vi "Lab Panel V4.89.vi"() -> ()   [LabVIEW 2013] (continued)
                            n1479 = local write "RESULT LAB05-2"(TRUE) -> ()
                            n1480 = local write "DISP LAB05-2"(w2793) -> ()
                          }
                        }
                      }
                      frame False {
                      }
                    }
                  }
                }
              }
            }
          }
          frame #6 {
            # "end test & close test files"
            n1481 = local read "MAIL SETTINGS"() -> (w2799:T7)
            n1482 = Unbundle(w2799) -> ("OUT SERVER ADDRESS"=w2798:string, "FROM ACCOUNT"=w2797:string)  [unwired: 5 out]
            n1483 = stacked-sequence {
              tunnel: w2809 -> [_ _ _ _ _ _ _ _ _ _]
              tunnel: w2810 -> [_ _ _ _ _ _ _ _ _ _]
              tunnel: w2808 -> [_ _ _ _ _ _ _ _ _ _]
              tunnel: w2807 -> [_ _ _ _ _ _ _ _ _ _]
              tunnel: w2806 -> [_ _ _ _ _ _ _ _ _ _]
              tunnel: w2805 -> [_ _ _ _ _ _ _ _ _ _]
              tunnel: w2804 -> [_ _ _ _ _ _ _ _ _ _]
              tunnel: w2803 -> [_ _ _ _ _ _ _ _ _ _]
              tunnel: w2802 -> [_ _ _ _ _ _ _ _ _ _]
              tunnel: w2801 -> [_ _ _ _ _ _ _ _ _ _]
              tunnel: w2798 -> [w2814 w2866 w2914 w2961 w3008 w3055 w3102 w3149 w3196 w3243]
              tunnel: w2797 -> [w2813 w2865 w2913 w2960 w3007 w3054 w3101 w3148 w3195 w3242]
              tunnel: "Mail Test File To:" -> [w2812 w2864 w2912 w2959 w3006 w3053 w3100 w3147 w3194 w3241]
              tunnel: "Mail Test Fail" -> [w2811 w2863 w2911 w2958 w3005 w3052 w3099 w3146 w3193 w3240]
              frame #0 {
                # "LAB01-1"
                n1484 = local read "DISP LAB01-1"() -> (w2818:T4)
                n1485 = local read "run lab01-1"() -> (w2815:bool)
                n1486 = local read "TDMS LAB01-1"() -> (w2816:refnum<k34>)
                n1487 = Unbundle(w2818) -> ("CYCLE"=w2819:dbl, "STATUS"=w2817:string)  [unwired: 1 out]
                n1488 = case shown="True" w2815 {
                  tunnel: w2819 -> [_ w2825]
                  tunnel: w2818 -> [_ w2827]
                  tunnel: w2817 -> [_ w2824]
                  tunnel: w2816 -> [_ w2826]
                  tunnel: w2814 -> [_ w2823]
                  tunnel: w2813 -> [_ w2822]
                  tunnel: w2812 -> [_ w2821]
                  tunnel: w2811 -> [_ w2820]
                  frame False {
                  }
                  frame True {
                    n1489 = Not Equal?(x=w2824, y="RUN") -> (x != y?=w2828:bool)
                    n1490 = Greater?(x=w2825, y=2.0) -> (0:w2830:bool)
                    n1491 = And(x=w2830, y=w2828) -> (x .and. y?=w2829:bool)
                    n1492 = case shown="True" w2829 {
                      tunnel: w2827 -> [_ w2840]
                      tunnel: w2826 -> [_ w2839]
                      tunnel: w2825 -> [_ w2838]
                      tunnel: w2824 -> [_ w2837]
                      tunnel: w2823 -> [_ w2836]
                      tunnel: w2822 -> [_ w2835]
                      tunnel: w2821 -> [_ w2834]
                      tunnel: w2820 -> [_ w2833]
                      frame False {
                      }
                      frame True {
                        n1493 = stacked-sequence {
                          tunnel: w2840 -> [w2844 _ _]
                          tunnel: w2839 -> [_ w2846 _]
                          tunnel: w2838 -> [_ _ _]
                          tunnel: w2837 -> [_ _ w2852]
                          tunnel: w2836 -> [_ _ w2851]
                          tunnel: w2835 -> [_ _ w2850]
                          tunnel: w2834 -> [_ _ w2849]
                          tunnel: w2833 -> [_ _ w2848]
                          frame #0 {
                            w2841 = FALSE
                            n1494 = local write "mail control"("END") -> ()
                            n1495 = Bundle(cluster=w2844) -> (w2843:T4)  [unwired: 3 in]
                            n1496 = local write "DISP LAB01-1"(w2843) -> ()
                            n1497 = local write "O/I  LAB01-1"(w2841) -> ()
                            n1498 = local write "run lab01-1"(w2841) -> ()
                            n1499 = local write "RUN LAB01-1"(w2841) -> ()
                          }
                          frame #1 {
                            n1500 = TDMS Close(11:w2846) -> (0:w2845:errorcluster)  [unwired: 1 in, 1 out]
                            n1501 = local write "data file error"(w2845) -> ()
                          }
                          frame #2 {
                            n1502 = stacked-sequence {
                              tunnel: "LAB01-1" -> [w2854 w2856 _]
                              tunnel: w2852 -> [_ w2862 _]
                              tunnel: w2851 -> [_ w2861 _]
                              tunnel: w2850 -> [_ w2860 _]
                              tunnel: w2849 -> [_ w2859 _]
                              tunnel: w2848 -> [_ w2858 _]
                              frame #0 {
                                n1503 = call "sub vi - defrag tdms v1.vi"("panel id"=w2854) -> ("error out"=w2853:errorcluster)  [unwired: 10 in]
                                n1504 = local write "data file error"(w2853) -> ()
                              }
                              frame #1 {
                                n1505 = Bundle("STATUS"=w2862, "OUT SERVER ADDRESS"=w2861, "FROM ACCOUNT"=w2860, "Mail Test File To:"=w2859, "Mail Test Fail"=w2858) -> (w2855:T25)  [unwired: 1 in]
                                n1506 = call "Save data file (pass-fail) v5.vi"("Input Cluster"=w2855, "panel id"=w2856) -> ("network file save error"=w2857:errorcluster)  [unwired: 8 in, 1 out]
                                n1507 = local write "data file error"(w2857) -> ()
                              }
                              frame #2 {
                              }
                            }
                          }
                        }
                      }
                    }
                  }
                }
              }
              frame #1 {
                # "LAB01-2"
                n1508 = local read "run lab01-2"() -> (w2867:bool)
                n1509 = case shown="True" w2867 {
                  tunnel: w2866 -> [_ w2871]
                  tunnel: w2865 -> [_ w2870]
                  tunnel: w2864 -> [_ w2869]
                  tunnel: w2863 -> [_ w2868]
                  frame False {
                  }
                  frame True {
                    n1510 = local read "DISP LAB01-2"() -> (w2879:T4)
                    n1511 = local read "TDMS LAB01-2"() -> (w2878:refnum<k34>)
                    n1512 = Unbundle(w2879) -> ("CYCLE"=w2873:dbl, "STATUS"=w2872:string)  [unwired: 1 out]
                    n1513 = Not Equal?(x=w2872, y="RUN") -> (x != y?=w2875:bool)
                    n1514 = Greater?(x=w2873, y=2.0) -> (0:w2876:bool)
                    n1515 = And(x=w2876, y=w2875) -> (x .and. y?=w2874:bool)
                    n1516 = case shown="True" w2874 {
                      tunnel: w2879 -> [_ w2888]
                      tunnel: w2878 -> [_ w2887]
                      tunnel: w2873 -> [_ w2886]
                      tunnel: w2872 -> [_ w2885]
                      tunnel: w2871 -> [_ w2884]
                      tunnel: w2870 -> [_ w2883]
                      tunnel: w2869 -> [_ w2882]
                      tunnel: w2868 -> [_ w2881]
                      frame False {
                      }
                      frame True {
                        n1517 = stacked-sequence {
                          tunnel: w2888 -> [w2891 _ _]
                          tunnel: w2887 -> [_ w2893 _]
                          tunnel: w2886 -> [_ _ _]
                          tunnel: w2885 -> [_ _ w2899]
                          tunnel: w2884 -> [_ _ w2898]
                          tunnel: w2883 -> [_ _ w2897]
                          tunnel: w2882 -> [_ _ w2896]
                          tunnel: w2881 -> [_ _ w2895]
                          frame #0 {
                            w2889 = FALSE
                            n1518 = local write "mail control"("END") -> ()
                            n1519 = Bundle(cluster=w2891) -> (w2892:T4)  [unwired: 3 in]
                            n1520 = local write "RUN LAB01-2"(w2889) -> ()
                            n1521 = local write "run lab01-2"(w2889) -> ()
                            n1522 = local write "O/I  LAB01-2"(w2889) -> ()
                            n1523 = local write "DISP LAB01-2"(w2892) -> ()
                          }
                          frame #1 {
                            n1524 = TDMS Close(11:w2893) -> (0:w2894:errorcluster)  [unwired: 1 in, 1 out]
                            n1525 = local write "data file error"(w2894) -> ()
                          }
                          frame #2 {
                            n1526 = stacked-sequence {
                              tunnel: "LAB01-2" -> [w2902 w2903]
                              tunnel: w2899 -> [_ w2908]
                              tunnel: w2898 -> [_ w2907]
                              tunnel: w2897 -> [_ w2906]
                              tunnel: w2896 -> [_ w2905]
                              tunnel: w2895 -> [_ w2904]
                              frame #0 {
                                n1527 = call "sub vi - defrag tdms v1.vi"("panel id"=w2902) -> ("error out"=w2901:errorcluster)  [unwired: 10 in]
                                n1528 = local write "data file error"(w2901) -> ()
                              }
                              frame #1 {
                                n1529 = Bundle("STATUS"=w2908, "OUT SERVER ADDRESS"=w2907, "FROM ACCOUNT"=w2906, "Mail Test File To:"=w2905, "Mail Test Fail"=w2904) -> (w2910:T25)  [unwired: 1 in]
                                n1530 = call "Save data file (pass-fail) v5.vi"("Input Cluster"=w2910, "panel id"=w2903) -> ("network file save error"=w2909:errorcluster)  [unwired: 8 in, 1 out]
                                n1531 = local write "data file error"(w2909) -> ()
                              }
                            }
                          }
                        }
                      }
                    }
                  }
                }
              }
              frame #2 {
                # "LAB02-1"
                n1532 = local read "run lab02-1"() -> (w2915:bool)
                n1533 = case shown="True" w2915 {
                  tunnel: w2914 -> [_ w2919]
                  tunnel: w2913 -> [_ w2918]
                  tunnel: w2912 -> [_ w2917]
                  tunnel: w2911 -> [_ w2916]
                  frame False {
                  }
                  frame True {
                    n1534 = local read "DISP LAB02-1"() -> (w2927:T4)
                    n1535 = Unbundle(w2927) -> ("CYCLE"=w2923:dbl, "STATUS"=w2920:string)  [unwired: 1 out]
                    n1536 = local read "TDMS LAB02-1"() -> (w2926:refnum<k34>)
                    n1537 = Not Equal?(x=w2920, y="RUN") -> (x != y?=w2922:bool)
                    n1538 = Greater?(x=w2923, y=2.0) -> (0:w2924:bool)
                    n1539 = And(x=w2924, y=w2922) -> (x .and. y?=w2921:bool)
                    n1540 = case shown="True" w2921 {
                      tunnel: w2927 -> [_ w2935]
                      tunnel: w2926 -> [_ w2934]
                      tunnel: w2920 -> [_ w2933]
                      tunnel: w2919 -> [_ w2932]
                      tunnel: w2918 -> [_ w2931]
                      tunnel: w2917 -> [_ w2930]
                      tunnel: w2916 -> [_ w2929]
                      frame False {
                      }
                      frame True {
                        n1541 = stacked-sequence {
                          tunnel: w2935 -> [w2938 _ _]
                          tunnel: w2934 -> [_ w2940 _]
                          tunnel: w2933 -> [_ _ w2946]
                          tunnel: w2932 -> [_ _ w2945]
                          tunnel: w2931 -> [_ _ w2944]
                          tunnel: w2930 -> [_ _ w2943]
                          tunnel: w2929 -> [_ _ w2942]
                          frame #0 {
                            w2936 = FALSE
                            n1542 = local write "mail control"("END") -> ()
                            n1543 = Bundle(cluster=w2938) -> (w2939:T4)  [unwired: 3 in]
                            n1544 = local write "O/I  LAB02-1"(w2936) -> ()
                            n1545 = local write "RUN LAB02-1"(w2936) -> ()
                            n1546 = local write "run lab02-1"(w2936) -> ()
                            n1547 = local write "DISP LAB02-1"(w2939) -> ()
                          }
                          frame #1 {
                            n1548 = TDMS Close(11:w2940) -> (0:w2941:errorcluster)  [unwired: 1 in, 1 out]
                            n1549 = local write "data file error"(w2941) -> ()
                          }
                          frame #2 {
                            n1550 = stacked-sequence {
                              tunnel: "LAB02-1" -> [w2949 w2956]
                              tunnel: w2946 -> [_ w2954]
                              tunnel: w2945 -> [_ w2953]
                              tunnel: w2944 -> [_ w2952]
                              tunnel: w2943 -> [_ w2951]
                              tunnel: w2942 -> [_ w2950]
                              frame #0 {
                                n1551 = call "sub vi - defrag tdms v1.vi"("panel id"=w2949) -> ("error out"=w2948:errorcluster)  [unwired: 10 in]
                                n1552 = local write "data file error"(w2948) -> ()
                              }
                              frame #1 {
                                n1553 = Bundle("STATUS"=w2954, "OUT SERVER ADDRESS"=w2953, "FROM ACCOUNT"=w2952, "Mail Test File To:"=w2951, "Mail Test Fail"=w2950) -> (w2955:T25)  [unwired: 1 in]
                                n1554 = call "Save data file (pass-fail) v5.vi"("Input Cluster"=w2955, "panel id"=w2956) -> ("network file save error"=w2957:errorcluster)  [unwired: 8 in, 1 out]
                                n1555 = local write "data file error"(w2957) -> ()
                              }
                            }
                          }
                        }
                      }
                    }
                  }
                }
              }
              frame #3 {
                # "LAB02-2"
                n1556 = local read "run lab02-2"() -> (w2962:bool)
                n1557 = case shown="True" w2962 {
                  tunnel: w2961 -> [_ w2966]
                  tunnel: w2960 -> [_ w2965]
                  tunnel: w2959 -> [_ w2964]
                  tunnel: w2958 -> [_ w2963]
                  frame False {
                  }
                  frame True {
                    n1558 = local read "DISP LAB02-2"() -> (w2974:T4)
                    n1559 = local read "TDMS LAB02-2"() -> (w2973:refnum<k34>)
                    n1560 = Unbundle(w2974) -> ("CYCLE"=w2970:dbl, "STATUS"=w2967:string)  [unwired: 1 out]
                    n1561 = Not Equal?(x=w2967, y="RUN") -> (x != y?=w2969:bool)
                    n1562 = Greater?(x=w2970, y=2.0) -> (0:w2971:bool)
                    n1563 = And(x=w2971, y=w2969) -> (x .and. y?=w2968:bool)
                    n1564 = case shown="True" w2968 {
                      tunnel: w2974 -> [_ w2982]
                      tunnel: w2973 -> [_ w2981]
                      tunnel: w2967 -> [_ w2980]
                      tunnel: w2966 -> [_ w2979]
                      tunnel: w2965 -> [_ w2978]
                      tunnel: w2964 -> [_ w2977]
                      tunnel: w2963 -> [_ w2976]
                      frame False {
                      }
                      frame True {
                        n1565 = stacked-sequence {
                          tunnel: w2982 -> [w2985 _ _]
                          tunnel: w2981 -> [_ w2987 _]
                          tunnel: w2980 -> [_ _ w2993]
                          tunnel: w2979 -> [_ _ w2992]
                          tunnel: w2978 -> [_ _ w2991]
                          tunnel: w2977 -> [_ _ w2990]
                          tunnel: w2976 -> [_ _ w2989]
                          frame #0 {
                            w2983 = FALSE
                            n1566 = local write "mail control"("END") -> ()
                            n1567 = Bundle(cluster=w2985) -> (w2986:T4)  [unwired: 3 in]
                            n1568 = local write "O/I  LAB02-2"(w2983) -> ()
                            n1569 = local write "run lab02-2"(w2983) -> ()
                            n1570 = local write "RUN LAB02-2"(w2983) -> ()
                            n1571 = local write "DISP LAB02-2"(w2986) -> ()
                          }
                          frame #1 {
                            n1572 = TDMS Close(11:w2987) -> (0:w2988:errorcluster)  [unwired: 1 in, 1 out]
                            n1573 = local write "data file error"(w2988) -> ()
                          }
                          frame #2 {
                            n1574 = stacked-sequence {
                              tunnel: "LAB02-2" -> [w2996 w3002]
                              tunnel: w2993 -> [_ w3001]
                              tunnel: w2992 -> [_ w3000]
                              tunnel: w2991 -> [_ w2999]
                              tunnel: w2990 -> [_ w2998]
                              tunnel: w2989 -> [_ w2997]
                              frame #0 {
                                n1575 = call "sub vi - defrag tdms v1.vi"("panel id"=w2996) -> ("error out"=w2995:errorcluster)  [unwired: 10 in]
                                n1576 = local write "data file error"(w2995) -> ()
                              }
                              frame #1 {
                                n1577 = Bundle("STATUS"=w3001, "OUT SERVER ADDRESS"=w3000, "FROM ACCOUNT"=w2999, "Mail Test File To:"=w2998, "Mail Test Fail"=w2997) -> (w3004:T25)  [unwired: 1 in]
                                n1578 = call "Save data file (pass-fail) v5.vi"("Input Cluster"=w3004, "panel id"=w3002) -> ("network file save error"=w3003:errorcluster)  [unwired: 8 in, 1 out]
                                n1579 = local write "data file error"(w3003) -> ()
                              }
                            }
                          }
                        }
                      }
                    }
                  }
                }
              }
              frame #4 {
                # "LAB03-1"
                n1580 = local read "run lab03-1"() -> (w3009:bool)
                n1581 = case shown="True" w3009 {
                  tunnel: w3008 -> [_ w3013]
                  tunnel: w3007 -> [_ w3012]
                  tunnel: w3006 -> [_ w3011]
                  tunnel: w3005 -> [_ w3010]
                  frame False {
                  }
                  frame True {
                    n1582 = local read "DISP LAB03-1"() -> (w3021:T4)
                    n1583 = local read "TDMS LAB03-1"() -> (w3020:refnum<k34>)
                    n1584 = Unbundle(w3021) -> ("CYCLE"=w3017:dbl, "STATUS"=w3014:string)  [unwired: 1 out]
                    n1585 = Not Equal?(x=w3014, y="RUN") -> (x != y?=w3016:bool)
                    n1586 = Greater?(x=w3017, y=2.0) -> (0:w3018:bool)
                    n1587 = And(x=w3018, y=w3016) -> (x .and. y?=w3015:bool)
                    n1588 = case shown="True" w3015 {
                      tunnel: w3021 -> [_ w3029]
                      tunnel: w3020 -> [_ w3028]
                      tunnel: w3014 -> [_ w3027]
                      tunnel: w3013 -> [_ w3026]
                      tunnel: w3012 -> [_ w3025]
                      tunnel: w3011 -> [_ w3024]
                      tunnel: w3010 -> [_ w3023]
                      frame False {
                      }
                      frame True {
                        n1589 = stacked-sequence {
                          tunnel: w3029 -> [w3032 _ _]
                          tunnel: w3028 -> [_ w3034 _]
                          tunnel: w3027 -> [_ _ w3040]
                          tunnel: w3026 -> [_ _ w3039]
                          tunnel: w3025 -> [_ _ w3038]
                          tunnel: w3024 -> [_ _ w3037]
                          tunnel: w3023 -> [_ _ w3036]
                          frame #0 {
                            w3030 = FALSE
                            n1590 = local write "mail control"("END") -> ()
                            n1591 = Bundle(cluster=w3032) -> (w3033:T4)  [unwired: 3 in]
                            n1592 = local write "O/I  LAB03-1"(w3030) -> ()
                            n1593 = local write "run lab03-1"(w3030) -> ()
                            n1594 = local write "RUN LAB03-1"(w3030) -> ()
                            n1595 = local write "DISP LAB03-1"(w3033) -> ()
                          }
                          frame #1 {
                            n1596 = TDMS Close(11:w3034) -> (0:w3035:errorcluster)  [unwired: 1 in, 1 out]
                            n1597 = local write "data file error"(w3035) -> ()
                          }
                          frame #2 {
                            n1598 = stacked-sequence {
                              tunnel: "LAB03-1" -> [w3043 w3049]
                              tunnel: w3040 -> [_ w3048]
                              tunnel: w3039 -> [_ w3047]
                              tunnel: w3038 -> [_ w3046]
                              tunnel: w3037 -> [_ w3045]
                              tunnel: w3036 -> [_ w3044]
                              frame #0 {
                                n1599 = call "sub vi - defrag tdms v1.vi"("panel id"=w3043) -> ("error out"=w3042:errorcluster)  [unwired: 10 in]
                                n1600 = local write "data file error"(w3042) -> ()
                              }
                              frame #1 {
                                n1601 = Bundle("STATUS"=w3048, "OUT SERVER ADDRESS"=w3047, "FROM ACCOUNT"=w3046, "Mail Test File To:"=w3045, "Mail Test Fail"=w3044) -> (w3051:T25)  [unwired: 1 in]
                                n1602 = call "Save data file (pass-fail) v5.vi"("Input Cluster"=w3051, "panel id"=w3049) -> ("network file save error"=w3050:errorcluster)  [unwired: 8 in, 1 out]
                                n1603 = local write "data file error"(w3050) -> ()
                              }
                            }
                          }
                        }
                      }
                    }
                  }
                }
              }
              frame #5 {
                # "LAB03-2"
                n1604 = local read "run lab03-2"() -> (w3056:bool)
                n1605 = case shown="True" w3056 {
                  tunnel: w3055 -> [_ w3060]
                  tunnel: w3054 -> [_ w3059]
                  tunnel: w3053 -> [_ w3058]
                  tunnel: w3052 -> [_ w3057]
                  frame False {
                  }
                  frame True {
                    n1606 = local read "DISP LAB03-2"() -> (w3068:T4)
                    n1607 = Unbundle(w3068) -> ("CYCLE"=w3064:dbl, "STATUS"=w3061:string)  [unwired: 1 out]
                    n1608 = local read "TDMS LAB03-2"() -> (w3067:refnum<k34>)
                    n1609 = Not Equal?(x=w3061, y="RUN") -> (x != y?=w3063:bool)
                    n1610 = Greater?(x=w3064, y=2.0) -> (0:w3065:bool)
                    n1611 = And(x=w3065, y=w3063) -> (x .and. y?=w3062:bool)
                    n1612 = case shown="True" w3062 {
                      tunnel: w3068 -> [_ w3076]
                      tunnel: w3067 -> [_ w3075]
                      tunnel: w3061 -> [_ w3074]
                      tunnel: w3060 -> [_ w3073]
                      tunnel: w3059 -> [_ w3072]
                      tunnel: w3058 -> [_ w3071]
                      tunnel: w3057 -> [_ w3070]
                      frame False {
                      }
                      frame True {
                        n1613 = stacked-sequence {
                          tunnel: w3076 -> [w3079 _ _]
                          tunnel: w3075 -> [_ w3081 _]
                          tunnel: w3074 -> [_ _ w3087]
                          tunnel: w3073 -> [_ _ w3086]
                          tunnel: w3072 -> [_ _ w3085]
                          tunnel: w3071 -> [_ _ w3084]
                          tunnel: w3070 -> [_ _ w3083]
                          frame #0 {
                            w3077 = FALSE
                            n1614 = local write "mail control"("END") -> ()
                            n1615 = Bundle(cluster=w3079) -> (w3080:T4)  [unwired: 3 in]
                            n1616 = local write "RUN LAB03-2"(w3077) -> ()
                            n1617 = local write "O/I  LAB03-2"(w3077) -> ()
                            n1618 = local write "DISP LAB03-2"(w3080) -> ()
                            n1619 = local write "run lab03-2"(w3077) -> ()
                          }
                          frame #1 {
                            n1620 = TDMS Close(11:w3081) -> (0:w3082:errorcluster)  [unwired: 1 in, 1 out]
                            n1621 = local write "data file error"(w3082) -> ()
                          }
                          frame #2 {
                            n1622 = stacked-sequence {
                              tunnel: "LAB03-2" -> [w3090 w3091]
                              tunnel: w3087 -> [_ w3096]
                              tunnel: w3086 -> [_ w3095]
                              tunnel: w3085 -> [_ w3094]
                              tunnel: w3084 -> [_ w3093]
                              tunnel: w3083 -> [_ w3092]
                              frame #0 {
                                n1623 = call "sub vi - defrag tdms v1.vi"("panel id"=w3090) -> ("error out"=w3089:errorcluster)  [unwired: 10 in]
                                n1624 = local write "data file error"(w3089) -> ()
                              }
                              frame #1 {
                                n1625 = Bundle("STATUS"=w3096, "OUT SERVER ADDRESS"=w3095, "FROM ACCOUNT"=w3094, "Mail Test File To:"=w3093, "Mail Test Fail"=w3092) -> (w3098:T25)  [unwired: 1 in]
                                n1626 = call "Save data file (pass-fail) v5.vi"("Input Cluster"=w3098, "panel id"=w3091) -> ("network file save error"=w3097:errorcluster)  [unwired: 8 in, 1 out]
                                n1627 = local write "data file error"(w3097) -> ()
                              }
                            }
                          }
                        }
                      }
                    }
                  }
                }
              }
              frame #6 {
                # "LAB04-1"
                n1628 = local read "run lab04-1"() -> (w3103:bool)
                n1629 = case shown="True" w3103 {
                  tunnel: w3102 -> [_ w3107]
                  tunnel: w3101 -> [_ w3106]
                  tunnel: w3100 -> [_ w3105]
                  tunnel: w3099 -> [_ w3104]
                  frame False {
                  }
                  frame True {
                    n1630 = local read "DISP LAB04-1"() -> (w3115:T4)
                    n1631 = Unbundle(w3115) -> ("CYCLE"=w3111:dbl, "STATUS"=w3108:string)  [unwired: 1 out]
                    n1632 = local read "TDMS LAB04-1"() -> (w3114:refnum<k34>)
                    n1633 = Not Equal?(x=w3108, y="RUN") -> (x != y?=w3110:bool)
                    n1634 = Greater?(x=w3111, y=2.0) -> (0:w3112:bool)
                    n1635 = And(x=w3112, y=w3110) -> (x .and. y?=w3109:bool)
                    n1636 = case shown="True" w3109 {
                      tunnel: w3115 -> [_ w3123]
                      tunnel: w3114 -> [_ w3122]
                      tunnel: w3108 -> [_ w3121]
                      tunnel: w3107 -> [_ w3120]
                      tunnel: w3106 -> [_ w3119]
                      tunnel: w3105 -> [_ w3118]
                      tunnel: w3104 -> [_ w3117]
                      frame False {
                      }
                      frame True {
                        n1637 = stacked-sequence {
                          tunnel: w3123 -> [w3126 _ _]
                          tunnel: w3122 -> [_ w3128 _]
                          tunnel: w3121 -> [_ _ w3134]
                          tunnel: w3120 -> [_ _ w3133]
                          tunnel: w3119 -> [_ _ w3132]
                          tunnel: w3118 -> [_ _ w3131]
                          tunnel: w3117 -> [_ _ w3130]
                          frame #0 {
                            w3124 = FALSE
                            n1638 = local write "mail control"("END") -> ()
                            n1639 = Bundle(cluster=w3126) -> (w3127:T4)  [unwired: 3 in]
                            n1640 = local write "RUN LAB04-1"(w3124) -> ()
                            n1641 = local write "O/I  LAB04-1"(w3124) -> ()
                            n1642 = local write "run lab04-1"(w3124) -> ()
                            n1643 = local write "DISP LAB04-1"(w3127) -> ()
                          }
                          frame #1 {
                            n1644 = TDMS Close(11:w3128) -> (0:w3129:errorcluster)  [unwired: 1 in, 1 out]
                            n1645 = local write "data file error"(w3129) -> ()
                          }
                          frame #2 {
                            n1646 = stacked-sequence {
                              tunnel: "LAB04-1" -> [w3137 w3138]
                              tunnel: w3134 -> [_ w3143]
                              tunnel: w3133 -> [_ w3142]
                              tunnel: w3132 -> [_ w3141]
                              tunnel: w3131 -> [_ w3140]
                              tunnel: w3130 -> [_ w3139]
                              frame #0 {
                                n1647 = call "sub vi - defrag tdms v1.vi"("panel id"=w3137) -> ("error out"=w3136:errorcluster)  [unwired: 10 in]
                                n1648 = local write "data file error"(w3136) -> ()
                              }
                              frame #1 {
                                n1649 = Bundle("STATUS"=w3143, "OUT SERVER ADDRESS"=w3142, "FROM ACCOUNT"=w3141, "Mail Test File To:"=w3140, "Mail Test Fail"=w3139) -> (w3145:T25)  [unwired: 1 in]
                                n1650 = call "Save data file (pass-fail) v5.vi"("Input Cluster"=w3145, "panel id"=w3138) -> ("network file save error"=w3144:errorcluster)  [unwired: 8 in, 1 out]
                                n1651 = local write "data file error"(w3144) -> ()
                              }
                            }
                          }
                        }
                      }
                    }
                  }
                }
              }
              frame #7 {
                # "LAB04-2"
                n1652 = local read "run lab04-2"() -> (w3150:bool)
                n1653 = case shown="True" w3150 {
                  tunnel: w3149 -> [_ w3154]
                  tunnel: w3148 -> [_ w3153]
                  tunnel: w3147 -> [_ w3152]
                  tunnel: w3146 -> [_ w3151]
                  frame False {
                  }
                  frame True {
                    n1654 = local read "DISP LAB04-2"() -> (w3162:T4)
                    n1655 = Unbundle(w3162) -> ("CYCLE"=w3158:dbl, "STATUS"=w3155:string)  [unwired: 1 out]
                    n1656 = Not Equal?(x=w3155, y="RUN") -> (x != y?=w3157:bool)
                    n1657 = local read "TDMS LAB04-2"() -> (w3161:refnum<k34>)
                    n1658 = Greater?(x=w3158, y=2.0) -> (0:w3159:bool)
                    n1659 = And(x=w3159, y=w3157) -> (x .and. y?=w3156:bool)
                    n1660 = case shown="True" w3156 {
                      tunnel: w3162 -> [_ w3170]
                      tunnel: w3161 -> [_ w3169]
                      tunnel: w3155 -> [_ w3168]
                      tunnel: w3154 -> [_ w3167]
                      tunnel: w3153 -> [_ w3166]
                      tunnel: w3152 -> [_ w3165]
                      tunnel: w3151 -> [_ w3164]
                      frame False {
                      }
                      frame True {
                        n1661 = stacked-sequence {
                          tunnel: w3170 -> [w3173 _ _]
                          tunnel: w3169 -> [_ w3175 _]
                          tunnel: w3168 -> [_ _ w3181]
                          tunnel: w3167 -> [_ _ w3180]
                          tunnel: w3166 -> [_ _ w3179]
                          tunnel: w3165 -> [_ _ w3178]
                          tunnel: w3164 -> [_ _ w3177]
                          frame #0 {
                            w3171 = FALSE
                            n1662 = local write "mail control"("END") -> ()
                            n1663 = Bundle(cluster=w3173) -> (w3174:T4)  [unwired: 3 in]
                            n1664 = local write "O/I  LAB04-2"(w3171) -> ()
                            n1665 = local write "RUN LAB04-2"(w3171) -> ()
                            n1666 = local write "run lab04-2"(w3171) -> ()
                            n1667 = local write "DISP LAB04-2"(w3174) -> ()
                          }
                          frame #1 {
                            n1668 = TDMS Close(11:w3175) -> (0:w3176:errorcluster)  [unwired: 1 in, 1 out]
                            n1669 = local write "data file error"(w3176) -> ()
                          }
                          frame #2 {
                            n1670 = stacked-sequence {
                              tunnel: "LAB04-2" -> [w3184 w3185]
                              tunnel: w3181 -> [_ w3190]
                              tunnel: w3180 -> [_ w3189]
                              tunnel: w3179 -> [_ w3188]
                              tunnel: w3178 -> [_ w3187]
                              tunnel: w3177 -> [_ w3186]
                              frame #0 {
                                n1671 = call "sub vi - defrag tdms v1.vi"("panel id"=w3184) -> ("error out"=w3183:errorcluster)  [unwired: 10 in]
                                n1672 = local write "data file error"(w3183) -> ()
                              }
                              frame #1 {
                                n1673 = Bundle("STATUS"=w3190, "OUT SERVER ADDRESS"=w3189, "FROM ACCOUNT"=w3188, "Mail Test File To:"=w3187, "Mail Test Fail"=w3186) -> (w3192:T25)  [unwired: 1 in]
                                n1674 = call "Save data file (pass-fail) v5.vi"("Input Cluster"=w3192, "panel id"=w3185) -> ("network file save error"=w3191:errorcluster)  [unwired: 8 in, 1 out]
                                n1675 = local write "data file error"(w3191) -> ()
                              }
                            }
                          }
                        }
                      }
                    }
                  }
                }
              }
              frame #8 {
                # "LAB05-1"
                n1676 = local read "run lab05-1"() -> (w3197:bool)
                n1677 = case shown="True" w3197 {
                  tunnel: w3196 -> [_ w3201]
                  tunnel: w3195 -> [_ w3200]
                  tunnel: w3194 -> [_ w3199]
                  tunnel: w3193 -> [_ w3198]
                  frame False {
                  }
                  frame True {
                    n1678 = local read "DISP LAB05-1"() -> (w3209:T4)
                    n1679 = Unbundle(w3209) -> ("CYCLE"=w3205:dbl, "STATUS"=w3202:string)  [unwired: 1 out]
                    n1680 = Not Equal?(x=w3202, y="RUN") -> (x != y?=w3204:bool)
                    n1681 = local read "TDMS LAB05-1"() -> (w3208:refnum<k34>)
                    n1682 = Greater?(x=w3205, y=2.0) -> (0:w3206:bool)
                    n1683 = And(x=w3206, y=w3204) -> (x .and. y?=w3203:bool)
                    n1684 = case shown="True" w3203 {
                      tunnel: w3209 -> [_ w3217]
                      tunnel: w3208 -> [_ w3216]
                      tunnel: w3202 -> [_ w3215]
                      tunnel: w3201 -> [_ w3214]
                      tunnel: w3200 -> [_ w3213]
                      tunnel: w3199 -> [_ w3212]
                      tunnel: w3198 -> [_ w3211]
                      frame False {
                      }
                      frame True {
                        n1685 = stacked-sequence {
                          tunnel: w3217 -> [w3220 _ _]
                          tunnel: w3216 -> [_ w3222 _]
                          tunnel: w3215 -> [_ _ w3228]
                          tunnel: w3214 -> [_ _ w3227]
                          tunnel: w3213 -> [_ _ w3226]
                          tunnel: w3212 -> [_ _ w3225]
                          tunnel: w3211 -> [_ _ w3224]
                          frame #0 {
                            w3218 = FALSE
                            n1686 = local write "mail control"("END") -> ()
                            n1687 = Bundle(cluster=w3220) -> (w3221:T4)  [unwired: 3 in]
                            n1688 = local write "O/I  LAB05-1"(w3218) -> ()
                            n1689 = local write "RUN LAB05-1"(w3218) -> ()
                            n1690 = local write "run lab05-1"(w3218) -> ()
                            n1691 = local write "DISP LAB05-1"(w3221) -> ()
                          }
                          frame #1 {
                            n1692 = TDMS Close(11:w3222) -> (0:w3223:errorcluster)  [unwired: 1 in, 1 out]
                            n1693 = local write "data file error"(w3223) -> ()
                          }
                          frame #2 {
                            n1694 = stacked-sequence {
                              tunnel: "LAB05-1" -> [w3231 w3237]
                              tunnel: w3228 -> [_ w3236]
                              tunnel: w3227 -> [_ w3235]
                              tunnel: w3226 -> [_ w3234]
                              tunnel: w3225 -> [_ w3233]
                              tunnel: w3224 -> [_ w3232]
                              frame #0 {
                                n1695 = call "sub vi - defrag tdms v1.vi"("panel id"=w3231) -> ("error out"=w3230:errorcluster)  [unwired: 10 in]
                                n1696 = local write "data file error"(w3230) -> ()
                              }
                              frame #1 {
                                n1697 = Bundle("STATUS"=w3236, "OUT SERVER ADDRESS"=w3235, "FROM ACCOUNT"=w3234, "Mail Test File To:"=w3233, "Mail Test Fail"=w3232) -> (w3239:T25)  [unwired: 1 in]
                                n1698 = call "Save data file (pass-fail) v5.vi"("Input Cluster"=w3239, "panel id"=w3237) -> ("network file save error"=w3238:errorcluster)  [unwired: 8 in, 1 out]
                                n1699 = local write "data file error"(w3238) -> ()
                              }
                            }
                          }
                        }
                      }
                    }
                  }
                }
              }
              frame #9 {
                # "LAB05-2"
                n1700 = local read "run lab05-2"() -> (w3244:bool)
                n1701 = case shown="True" w3244 {
                  tunnel: w3243 -> [_ w3248]
                  tunnel: w3242 -> [_ w3247]
                  tunnel: w3241 -> [_ w3246]
                  tunnel: w3240 -> [_ w3245]
                  frame False {
                  }
                  frame True {
                    n1702 = local read "DISP LAB05-2"() -> (w3256:T4)
                    n1703 = Unbundle(w3256) -> ("CYCLE"=w3252:dbl, "STATUS"=w3249:string)  [unwired: 1 out]
                    n1704 = Not Equal?(x=w3249, y="RUN") -> (x != y?=w3251:bool)
                    n1705 = local read "TDMS LAB05-2"() -> (w3255:refnum<k34>)
                    n1706 = Greater?(x=w3252, y=2.0) -> (0:w3253:bool)
                    n1707 = And(x=w3253, y=w3251) -> (x .and. y?=w3250:bool)
                    n1708 = case shown="True" w3250 {
                      tunnel: w3256 -> [_ w3264]
                      tunnel: w3255 -> [_ w3263]
                      tunnel: w3249 -> [_ w3262]
                      tunnel: w3248 -> [_ w3261]
                      tunnel: w3247 -> [_ w3260]
                      tunnel: w3246 -> [_ w3259]
                      tunnel: w3245 -> [_ w3258]
                      frame False {
                      }
                      frame True {
                        n1709 = stacked-sequence {
                          tunnel: w3264 -> [w3267 _ _]
                          tunnel: w3263 -> [_ w3269 _]
                          tunnel: w3262 -> [_ _ w3275]
                          tunnel: w3261 -> [_ _ w3274]
                          tunnel: w3260 -> [_ _ w3273]
                          tunnel: w3259 -> [_ _ w3272]
                          tunnel: w3258 -> [_ _ w3271]
                          frame #0 {
                            w3265 = FALSE
                            n1710 = local write "mail control"("END") -> ()
                            n1711 = Bundle(cluster=w3267) -> (w3268:T4)  [unwired: 3 in]
                            n1712 = local write "RUN LAB05-2"(w3265) -> ()
                            n1713 = local write "O/I  LAB05-2"(w3265) -> ()
                            n1714 = local write "run lab05-2"(w3265) -> ()
                            n1715 = local write "DISP LAB05-2"(w3268) -> ()
                          }
                          frame #1 {
                            n1716 = TDMS Close(11:w3269) -> (0:w3270:errorcluster)  [unwired: 1 in, 1 out]
                            n1717 = local write "data file error"(w3270) -> ()
                          }
                          frame #2 {
                            n1718 = stacked-sequence {
                              tunnel: "LAB05-2" -> [w3278 w3284]
                              tunnel: w3275 -> [_ w3283]
                              tunnel: w3274 -> [_ w3282]
                              tunnel: w3273 -> [_ w3281]
                              tunnel: w3272 -> [_ w3280]
                              tunnel: w3271 -> [_ w3279]
                              frame #0 {
                                n1719 = call "sub vi - defrag tdms v1.vi"("panel id"=w3278) -> ("error out"=w3277:errorcluster)  [unwired: 10 in]
                                n1720 = local write "data file error"(w3277) -> ()
                              }
                              frame #1 {
                                n1721 = Bundle("STATUS"=w3283, "OUT SERVER ADDRESS"=w3282, "FROM ACCOUNT"=w3281, "Mail Test File To:"=w3280, "Mail Test Fail"=w3279) -> (w3286:T25)  [unwired: 1 in]
                                n1722 = call "Save data file (pass-fail) v5.vi"("Input Cluster"=w3286, "panel id"=w3284) -> ("network file save error"=w3285:errorcluster)  [unwired: 8 in, 1 out]
                                n1723 = local write "data file error"(w3285) -> ()
                              }
                            }
                          }
                        }
                      }
                    }
                  }
                }
              }
            }
            n1724 = local read "Network Directory"() -> (w2800:path)
            n1725 = global write "Global 1.vi" "Network Drive"(w2800) -> ()
          }
          frame #7 {
            # "disable functions"
            n1726 = stacked-sequence {
              tunnel: w3296 -> [w3310 _ w3367]
              tunnel: w3295 -> [w3305 _ w3366]
              tunnel: w3294 -> [w3304 _ w3365]
              tunnel: w3293 -> [w3302 _ w3364]
              tunnel: w3292 -> [w3303 _ w3363]
              tunnel: w3291 -> [_ w3327 w3362]
              tunnel: w3290 -> [_ w3328 w3361]
              tunnel: w3289 -> [_ w3329 w3360]
              tunnel: w3288 -> [_ w3330 w3359]
              tunnel: w3287 -> [_ w3331 w3358]
              frame #0 {
                n1727 = Select(t=2, s=w3302, f=0) -> (s? t:f=w3298:i32)
                n1728 = Select(t=2, s=w3304, f=0) -> (s? t:f=w3299:i32)
                n1729 = Select(t=2, s=w3303, f=0) -> (s? t:f=w3297:i32)
                n1730 = Select(t=2, s=w3310, f=0) -> (s? t:f=w3301:i32)
                n1731 = Select(t=2, s=w3305, f=0) -> (s? t:f=w3300:i32)
                n1732 = property on="SELECT LAB02-2" class="RadioBtnsControl (strict)"("DisabledEnum"=w3298) -> ()  [unwired: 2 in, 2 out]
                n1733 = property on="SELECT LAB02-1" class="RadioBtnsControl (strict)"("DisabledEnum"=w3299) -> ()  [unwired: 2 in, 2 out]
                n1734 = property on="SELECT LAB03-1" class="RadioBtnsControl (strict)"("DisabledEnum"=w3297) -> ()  [unwired: 2 in, 2 out]
                n1735 = property on="SELECT LAB01-1" class="RadioBtnsControl (strict)"("DisabledEnum"=w3301) -> ()  [unwired: 2 in, 2 out]
                n1736 = property on="SELECT LAB01-2" class="RadioBtnsControl (strict)"("DisabledEnum"=w3300) -> ()  [unwired: 2 in, 2 out]
                n1737 = Not(x=w3310) -> (.not. x?=w3311:bool)
                n1738 = property on="RESULT LAB01-1" class="Bool (strict)"("Visible"=w3311) -> ()  [unwired: 2 in, 2 out]
                n1739 = Not(x=w3305) -> (.not. x?=w3309:bool)
                n1740 = Not(x=w3304) -> (.not. x?=w3308:bool)
                n1741 = Not(x=w3302) -> (.not. x?=w3307:bool)
                n1742 = property on="RESULT LAB01-2" class="Bool (strict)"("Visible"=w3309) -> ()  [unwired: 2 in, 2 out]
                n1743 = Not(x=w3303) -> (.not. x?=w3306:bool)
                n1744 = property on="RESULT LAB02-1" class="Bool (strict)"("Visible"=w3308) -> ()  [unwired: 2 in, 2 out]
                n1745 = property on="RESULT LAB02-2" class="Bool (strict)"("Visible"=w3307) -> ()  [unwired: 2 in, 2 out]
                n1746 = property on="RESULT LAB03-1" class="Bool (strict)"("Visible"=w3306) -> ()  [unwired: 2 in, 2 out]
                n1747 = property on="SET LAB01-1" class="Clust (strict)"("DisabledEnum"=w3301) -> ()  [unwired: 2 in, 2 out]
                n1748 = property on="SET LAB01-2" class="Clust (strict)"("DisabledEnum"=w3300) -> ()  [unwired: 2 in, 2 out]
                n1749 = property on="SET LAB02-1" class="Clust (strict)"("DisabledEnum"=w3299) -> ()  [unwired: 2 in, 2 out]
                n1750 = property on="SET LAB02-2" class="Clust (strict)"("DisabledEnum"=w3298) -> ()  [unwired: 2 in, 2 out]
                n1751 = property on="SET LAB03-1" class="Clust (strict)"("DisabledEnum"=w3297) -> ()  [unwired: 2 in, 2 out]
                n1752 = property on="O/I  LAB01-1" class="Bool (strict)"("DisabledEnum"=w3301) -> ()  [unwired: 2 in, 2 out]
                n1753 = property on="O/I  LAB01-2" class="Bool (strict)"("DisabledEnum"=w3300) -> ()  [unwired: 2 in, 2 out]
                n1754 = property on="O/I  LAB02-1" class="Bool (strict)"("DisabledEnum"=w3299) -> ()  [unwired: 2 in, 2 out]
                n1755 = property on="O/I  LAB02-2" class="Bool (strict)"("DisabledEnum"=w3298) -> ()  [unwired: 2 in, 2 out]
                n1756 = property on="O/I  LAB03-1" class="Bool (strict)"("DisabledEnum"=w3297) -> ()  [unwired: 2 in, 2 out]
              }
              frame #1 {
                n1757 = Select(t=2, s=w3331, f=0) -> (s? t:f=w3322:i32)
                n1758 = Select(t=2, s=w3330, f=0) -> (s? t:f=w3323:i32)
                n1759 = Select(t=2, s=w3327, f=0) -> (s? t:f=w3326:i32)
                n1760 = Select(t=2, s=w3328, f=0) -> (s? t:f=w3325:i32)
                n1761 = Select(t=2, s=w3329, f=0) -> (s? t:f=w3324:i32)
                n1762 = property on="SELECT LAB05-2" class="RadioBtnsControl (strict)"("DisabledEnum"=w3322) -> ()  [unwired: 2 in, 2 out]
                n1763 = property on="SELECT LAB05-1" class="RadioBtnsControl (strict)"("DisabledEnum"=w3323) -> ()  [unwired: 2 in, 2 out]
                n1764 = property on="SELECT LAB03-2" class="RadioBtnsControl (strict)"("DisabledEnum"=w3326) -> ()  [unwired: 2 in, 2 out]
                n1765 = property on="SELECT LAB04-1" class="RadioBtnsControl (strict)"("DisabledEnum"=w3325) -> ()  [unwired: 2 in, 2 out]
                n1766 = property on="SELECT LAB04-2" class="RadioBtnsControl (strict)"("DisabledEnum"=w3324) -> ()  [unwired: 2 in, 2 out]
                n1767 = property on="SET LAB05-2" class="Clust (strict)"("DisabledEnum"=w3322) -> ()  [unwired: 2 in, 2 out]
                n1768 = property on="SET LAB05-1" class="Clust (strict)"("DisabledEnum"=w3323) -> ()  [unwired: 2 in, 2 out]
                n1769 = property on="SET LAB03-2" class="Clust (strict)"("DisabledEnum"=w3326) -> ()  [unwired: 2 in, 2 out]
                n1770 = property on="SET LAB04-1" class="Clust (strict)"("DisabledEnum"=w3325) -> ()  [unwired: 2 in, 2 out]
                n1771 = property on="SET LAB04-2" class="Clust (strict)"("DisabledEnum"=w3324) -> ()  [unwired: 2 in, 2 out]
                n1772 = property on="O/I  LAB05-2" class="Bool (strict)"("DisabledEnum"=w3322) -> ()  [unwired: 2 in, 2 out]
                n1773 = property on="O/I  LAB05-1" class="Bool (strict)"("DisabledEnum"=w3323) -> ()  [unwired: 2 in, 2 out]
                n1774 = property on="O/I  LAB04-1" class="Bool (strict)"("DisabledEnum"=w3325) -> ()  [unwired: 2 in, 2 out]
                n1775 = property on="O/I  LAB04-2" class="Bool (strict)"("DisabledEnum"=w3324) -> ()  [unwired: 2 in, 2 out]
